vi "IO Control.vi"(8 "error in (no error)":errorcluster, 11 "Node Ptr":T1 format="%.0x") -> (0 "error out":errorcluster)   [LabVIEW 2015, in "Diagnostics Addon System Explorer.lvlib"]
uses:
  Diagnostics Addon System Explorer.lvlib
  <vilib>/NI Veristand/Custom Device API/Custom Device Item Ref.ctl
  Shared/FG Action.ctl
  Shared/GUID Lookup.vi
  <vilib>/NI Veristand/Custom Device API/NI VeriStand - Set Item Property.vi
  <vilib>/NI Veristand/Custom Device API/Set Item Property (U32).vi
  <vilib>/NI Veristand/Custom Device API/NI VeriStand - Get Item Property.vi
  <vilib>/NI Veristand/Custom Device API/Get Item Property (U32).vi
  <vilib>/NI Veristand/Custom Device API/Custom Device API.lvlib
panel:
  in  "SHDocVw.IWebBrowser":refnum<k7>(container)
  in  "IO Control":i32(listbox)
  in  "Description":string
  out "Name":string
  in  "Header":cluster{"Section Name":string}={"Section Name"="Custom Device Item Settings"}
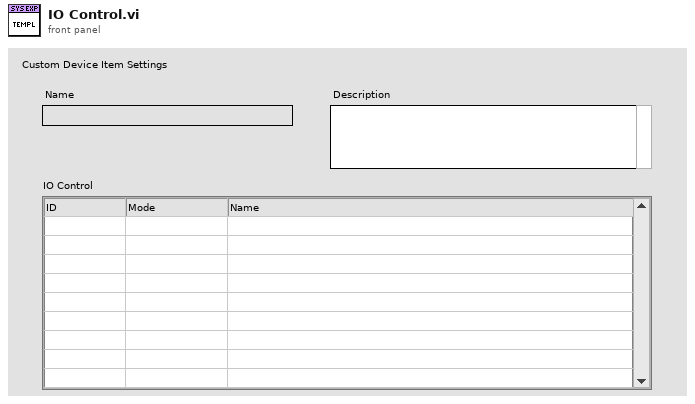
[diagram p1: front panel]
types:
  T1 = typedef "Custom Device API.lvlib/Custom Device Item Ref.ctl" = u64
  T2 = typedef "Diagnostics Addon System Explorer.lvlib/FG Action.ctl" = enum16{"Get", "Set"}
  T3 = typedef "Custom Device API.lvlib/Custom Device Item Info.ctl" = cluster{"Name":string, "Is Channel":bool, "GUID":string, "Is Waveform":bool}
  T4 = typedef "Custom Device API.lvlib/Custom Device Commands.ctl" = enum16{"Default", "Item renamed", "Shutdown", "Dynamic button pressed"}
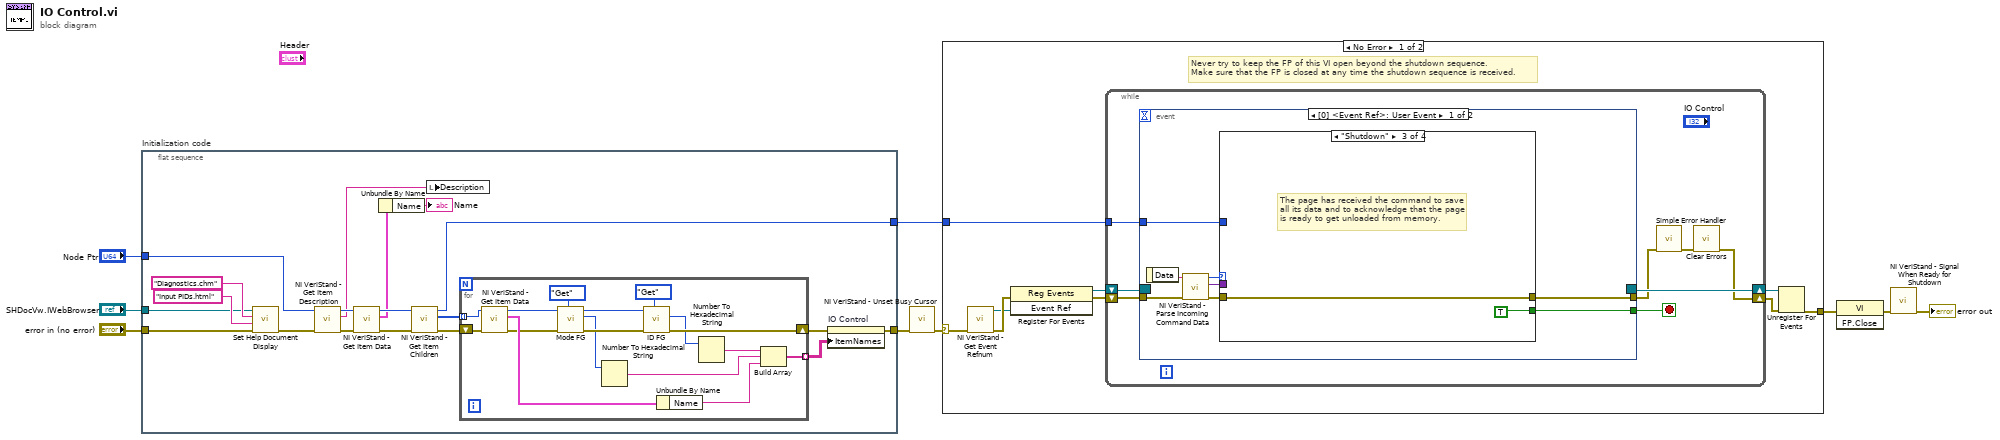
[diagram p0: block diagram]
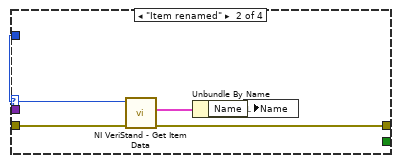
[diagram p3: hidden frame]
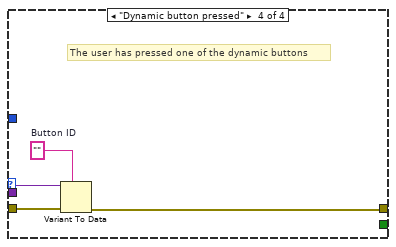
[diagram p4: hidden frame]
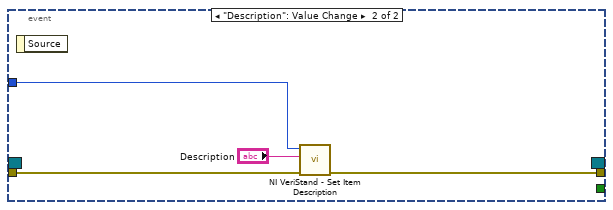
[diagram p5: hidden frame]
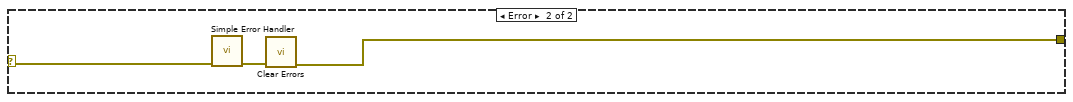
[diagram p6: hidden frame]
diagram:
  n1 = flat-sequence "Initialization code" {
    tunnel: "error in (no error)" -> [w21]
    tunnel: [w12] -> w6
    tunnel: [w14] -> w3
    tunnel: "Node Ptr" -> [w19]
    tunnel: "SHDocVw.IWebBrowser" -> [w18]
    frame #0 {
      n2 = call "Set Help Document Display.vi"("error in (no error)"=w21, "HTML File"="Input PIDs.html", "Main CHM File"="Diagnostics.chm", "SHDocVw.IWebBrowser2"=w18) -> ("error out"=w20:errorcluster)  [unwired: 7 in]
      n3 = call <vilib>:"NI VeriStand - Get Item Description.vi"("error in (no error)"=w20, "Item Ref in"=w19) -> ("error out"=w25:errorcluster, "Description"=w26:string, "Item Ref out"=w27:T1)  [unwired: 7 out]
      n4 = call <vilib>:"NI VeriStand - Get Item Data.vi"("error in (no error)"=w25, "Item Ref in"=w27) -> ("error out"=w17:errorcluster, "Item Info"=w24:T3, "Item Ref out"=w28:T1)  [unwired: 7 out]
      n5 = Unbundle By Name(w24) -> ("Name"=→"Name":string)
      n6 = call <vilib>:"NI VeriStand - Get Item Children.vi"("error in (no error)"=w17, "Item Ref in"=w28) -> ("error out"=w16:errorcluster, "Child Refs"=w15:T1[], "Item Ref out"=w14:T1)  [unwired: 6 in, 1 out]
      n7 = local write "Description"(w26) -> ()
      n8 = for {
        shift-right: [w36] -> w13
        shift-left: w16 -> [w44]
        tunnel: w15 -> [w43] mode=indexing
        tunnel: [w40] -> w11 mode=indexing
        n9 = call <vilib>:"NI VeriStand - Get Item Data.vi"("error in (no error)"=w44, "Item Ref in"=w43) -> ("error out"=w34:errorcluster, "Item Info"=w42:T3, "Item Ref out"=w32:T1)  [unwired: 7 out]
        n10 = call "Mode FG.vi"("Action"=FG_Action."Get", "error in (no error)"=w34, "Device Item Ref in"=w32) -> ("error out"=w33:errorcluster, "Mode"=w30:u32, "Device Item Ref out"=w31:T1)  [unwired: 6 in]
        n11 = Number To Hexadecimal String(2:w30) -> (0:w38:string)  [unwired: 1 in]
        n12 = call "ID FG.vi"("Action"=FG_Action."Get", "error in (no error)"=w33, "Device Item Ref in"=w31) -> ("error out"=w36:errorcluster, "ID"=w35:u32)  [unwired: 6 in, 1 out]
        n13 = Unbundle By Name(w42) -> ("Name"=w41:string)
        n14 = Number To Hexadecimal String(2:w35) -> (0:w39:string)  [unwired: 1 in]
        n15 = Build Array(w39, w38, w41) -> (w40:string[])
      }
      n16 = property on="IO Control" class="MCListbox (strict)"(error in=w13, "ItemNames"=w11) -> (error out=w12:errorcluster)  [unwired: 1 in, 1 out]
    }
  }
  n17 = call <vilib>:"NI VeriStand - Unset Busy Cursor.vi"("error in (no error)"=w6) -> ("error out"=w5:errorcluster)  [unwired: 10 out]
  n18 = case shown="No Error" w5 {
    selector: w5 -> [w45 w88]
    tunnel: [w50 w86] -> w9
    tunnel: w3 -> [w46 _]
    frame No Error {
      # "Never try to keep the FP of this VI open beyond the shutdown sequence.\nMake sure that the FP is closed at any time the shutdown sequence is received."
      n19 = call <vilib>:"NI VeriStand - Get Event Refnum.vi"("error in (no error)"=w45) -> ("error out"=w53:errorcluster, "Event Ref"=w49:refnum<user-event>)  [unwired: 9 out]
      n20 = register-events(error in=w53, w49) -> (reference out=w47:refnum<event-registration>, error out=w48:errorcluster)  [unwired: 1 in]
      n21 = while {
        tunnel: w46 -> [w57]
        shift-right: [w54] -> w51
        shift-left: w48 -> [w60]
        shift-right: [w61] -> w52
        shift-left: w47 -> [w59]
        stop <- w58 stop-if-true
        n22 = event shown="[0] <Event Ref>: User Event" {
          selector: w59 -> [_ _]
          dyn-events: [_ _] -> w61
          timeout: _ -> [_ _]
          tunnel: w60 -> [w69 w84]
          tunnel: [w65 _] -> w58
          tunnel: [w64 w83] -> w56
          tunnel: w57 -> [w63 w85]
          event User Event {
            n23 = event-data() -> ("Data"=w68:string)  [unwired: 1 out]
            n24 = call <vilib>:"NI VeriStand - Parse Incoming Command Data.vi"("error in (no error)"=w69, "Incoming data"=w68) -> ("error out"=w67:errorcluster, "Outgoing data"=w62:variant, "Action"=w66:T4)  [unwired: 7 out]
            n25 = case shown="\"Shutdown\"" w66 {
              tunnel: w67 -> [w70 w75 w76 w81]
              tunnel: [_ _ TRUE _] -> w65
              tunnel: [w70 w72 w76 w78] -> w64
              tunnel: w63 -> [_ w74 _ _]
              tunnel: w62 -> [_ _ _ w80]
              frame "Default", Default {
              }
              frame "Item renamed" {
                n26 = call <vilib>:"NI VeriStand - Get Item Data.vi"("error in (no error)"=w75, "Item Ref in"=w74) -> ("error out"=w72:errorcluster, "Item Info"=w73:T3)  [unwired: 8 out]
                n27 = Unbundle By Name(w73) -> ("Name"=w71:string)
                n28 = local write "Name"(w71) -> ()
              }
              frame "Shutdown" {
                # "The page has received the command to save all its data and to acknowledge that the page is ready to get unloaded from memory."
              }
              frame "Dynamic button pressed" {
                w79 = ""  # Button ID
                # "The user has pressed one of the dynamic buttons"
                n29 = Variant To Data(error in=w81, type=w79, Variant=w80) -> (error out=w78:errorcluster)  [unwired: 1 out]
              }
            }
          }
          event "Description": Value Change {
            n30 = event-data() -> ()  [unwired: 2 out]
            n31 = call <vilib>:"NI VeriStand - Set Item Description.vi"("error in (no error)"=w84, "Description"="Description", "Item Ref in"=w85) -> ("error out"=w83:errorcluster)  [unwired: 8 out]
          }
        }
        n32 = call <vilib>:"Simple Error Handler.vi"("error in (no error)"=w56) -> ("error out"=w55:errorcluster)  [unwired: 1 in, 7 out]
        n33 = call <vilib>:"Clear Errors.vi"("error in (no error)"=w55) -> ("error out"=w54:errorcluster)  [unwired: 1 in, 5 out]
      }
      n34 = Unregister For Events(event registration refnum=w52, error in=w51) -> (error out=w50:errorcluster)
    }
    frame Error {
      n35 = call <vilib>:"Simple Error Handler.vi"("error in (no error)"=w88) -> ("error out"=w87:errorcluster)  [unwired: 1 in, 7 out]
      n36 = call <vilib>:"Clear Errors.vi"("error in (no error)"=w87) -> ("error out"=w86:errorcluster)  [unwired: 1 in, 5 out]
    }
  }
  n37 = invoke class="VI" method="FP.Close"(error in=w9) -> (error out=w8:errorcluster)  [unwired: 2 in, 2 out]
  n38 = call <vilib>:"NI VeriStand - Signal When Ready for Shutdown.vi"("error in (no error)"=w8) -> ("error out"=→"error out":errorcluster)  [unwired: 10 out]
